vi "sine_fit_test_ab.vi"() -> ()   [LabVIEW 2018]
uses:
  <vilib>/measure/NI_MABase.lvlib
panel:
  out "Fit Coefficients":dbl[](array[numeric]) format="%.3g"
  out "Compare Data and Fit":waveform(dbl)[](graph)
  in  "Offset":dbl
  in  "Fs":dbl
  in  "Phase":dbl
  in  "Samples":dbl
  in  "Frequency":dbl
  in  "Amplitude":dbl
  # "Amplitude"
  # "Phase Offset (deg)"
  # "Frequency"
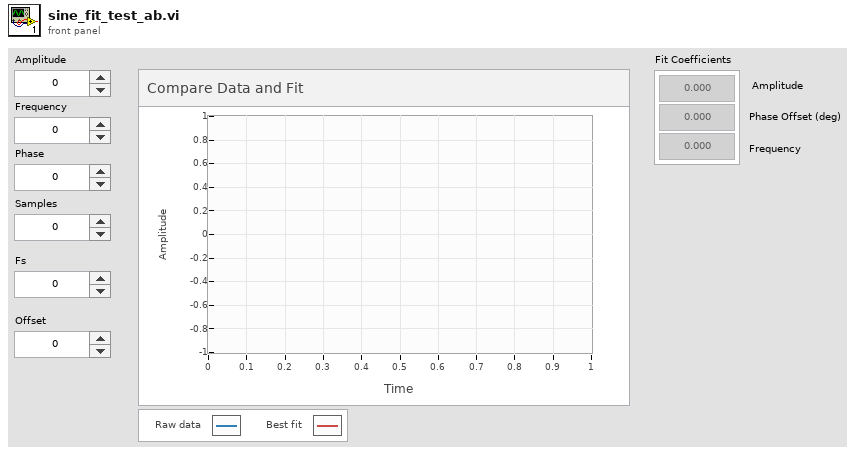
[diagram p1: front panel]
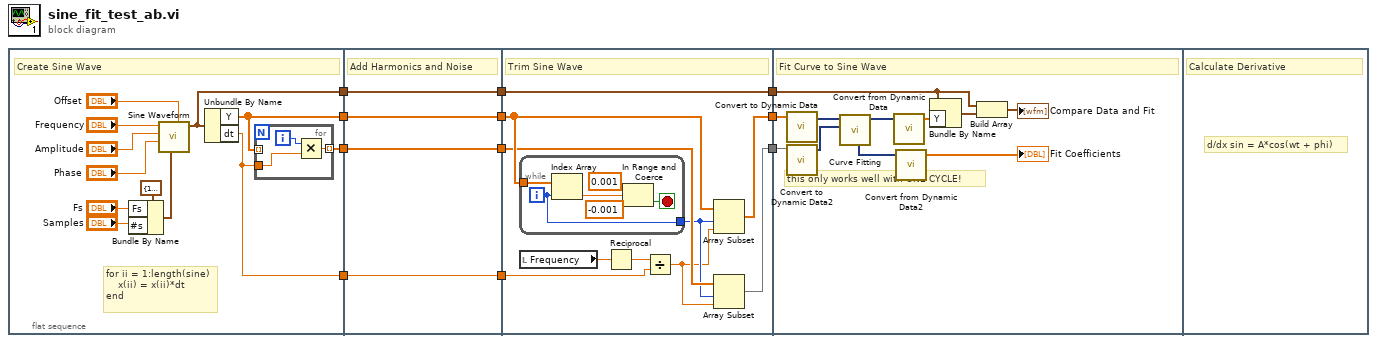
[diagram p0: block diagram]
diagram:
  n1 = flat-sequence {
    tunnel: [w15] -> w11
    tunnel: [w14] -> w10
    tunnel: [w13] -> w9
    tunnel: [w12] -> w2
    tunnel: w11 -> [w30]
    tunnel: [w30] -> w8
    tunnel: w10 -> [w29]
    tunnel: [w29] -> w6
    tunnel: w9 -> [w28]
    tunnel: [w28] -> w4
    tunnel: w2 -> [w27]
    tunnel: [w27] -> w1
    tunnel: w8 -> [w39]
    tunnel: [w35] -> w7
    tunnel: w6 -> [w34]
    tunnel: [w31] -> w5
    tunnel: w4 -> [w40]
    tunnel: [w40] -> w3
    tunnel: w1 -> [w36]
    tunnel: w7 -> [w57]
    tunnel: w5 -> [w55]
    tunnel: w3 -> [w50]
    frame #0 {
      # "for ii = 1:length(sine)\n    x(ii) = x(ii)*dt\nend"
      # "Create Sine Wave"
      n2 = Bundle By Name(cluster=cluster{"Fs":dbl, "#s":dbl} {"Fs"=1000.0, "#s"=1000.0} ("sampling info"), "Fs"="Fs", "#s"="Samples") -> (w17:cluster{"Fs":dbl, "#s":dbl})
      n3 = call <vilib>:"Sine Waveform.vi"("offset"="Offset", "sampling info"=w17, "phase"="Phase", "amplitude"="Amplitude", "frequency"="Frequency") -> ("signal out"=w13:waveform(dbl))  [unwired: 5 in, 1 out]
      n4 = Unbundle By Name(w13) -> ("Y"=w15:dbl[], "dt"=w12:dbl)
      n5 = for {
        tunnel: w12 -> [w26]
        tunnel: [w25] -> w14 mode=indexing
        tunnel: w15 -> [_] mode=indexing
        i -> [w24]
        n6 = Multiply(x=w24, y=w26) -> (x*y=w25:dbl)
      }
    }
    frame #1 {
      # "Add Harmonics and Noise"
    }
    frame #2 {
      # "Trim Sine Wave"
      n7 = while {
        tunnel: w39 -> [w44]
        tunnel: [w41] -> w33
        i -> [w41]
        stop <- w42 stop-if-true
        n8 = Index Array(array=w44, index=w41) -> (element=w43:dbl)
        n9 = In Range and Coerce(upper limit=0.001, x=w43, lower limit=-0.001) -> (In Range?=w42:bool)  [unwired: 1 out]
      }
      n10 = local read "Frequency"() -> (w38:dbl)
      n11 = Reciprocal(x=w38) -> (1/x=w37:dbl)
      n12 = Divide(x=w37, y=w36) -> (x/y=w32:dbl)
      n13 = Array Subset(array=w39, index=w33, length=w32) -> (w35:dbl[])
      n14 = Array Subset(array=w34, index=w33, length=w32) -> (w31:dbl[])
    }
    frame #3 {
      # "this only works well with ONE CYCLE!"
      # "Fit Curve to Sine Wave"
      n15 = call "Convert to Dynamic Data"("Array"=w57) -> ("Dynamic Data Type"=w56:dynamicdata)  [unwired: 3 in]
      n16 = call "Convert to Dynamic Data2"("Array"=w55) -> ("Dynamic Data Type"=w54:dynamicdata)  [unwired: 3 in]
      n17 = call "Curve Fitting"("Locations"=w54, "Signals"=w56) -> ("best fit"=w53:dynamicdata, "non-linear coefficients"=w48:dynamicdata)  [unwired: 5 in, 3 out]
      n18 = call "Convert from Dynamic Data"("Dynamic Data Type"=w53) -> ("Array"=w51:dbl[])  [unwired: 3 in]
      n19 = call "Convert from Dynamic Data2"("Dynamic Data Type"=w48) -> ("Array"=→"Fit Coefficients":dbl[])  [unwired: 3 in]
      n20 = Bundle By Name(cluster=w50, "Y"=w51) -> (w49:waveform(dbl))
      n21 = Build Array(w50, w49) -> (→"Compare Data and Fit":waveform(dbl)[])
    }
    frame #4 {
      # "d/dx sin = A*cos(wt + phi)"
      # "Calculate Derivative"
    }
  }
